vi "process safe state.vi"(8 "error in":errorcluster, 9 "result allocation":T1, 10 "parameters":T1, 11 "AppStateMachine runtime in":refnum<class "AppStateMachine runtime.lvclass">) -> (0 "error out":errorcluster, 1 "results":T1, 2 "parameter allocation":T1, 3 "AppStateMachine runtime out":refnum<class "AppStateMachine runtime.lvclass">)   [LabVIEW 2017, in "AppStateMachine runtime.lvclass"]
doc: "Provides an interface for information processing by a module when in a safe state. This interface simply calls the normal processing function. However, if child modules need to have custom logic during safe-state operation, this can be implemented here.\nNI Tag Bus Module Framework 1.0.2.34\nNI Systems Engineering"
uses:
  AppStateMachine runtime.lvclass
  <vilib>/NI/Tag Bus/table/data table.ctl
  State.ctl
  StateId.ctl
  LED_Color.ctl
  AppStateMachine runtime.lvclass/AppStateMachine runtime.ctl
  <vilib>/NI/Tag Bus/table/data table.lvlib
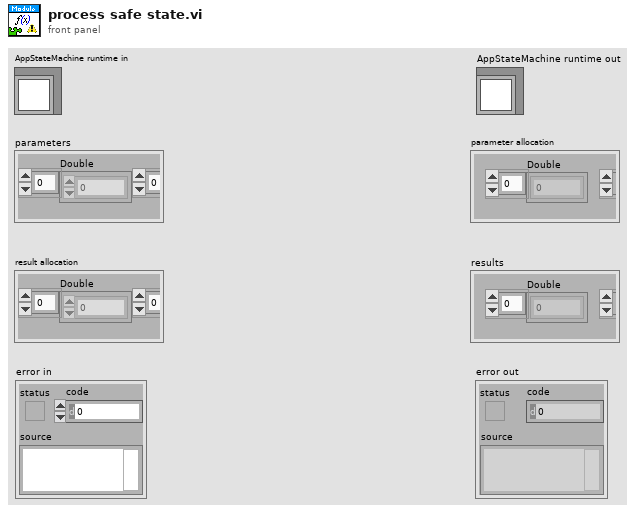
[diagram p1: front panel]
types:
  T1 = typedef "tag bus.lvlib/data table.lvlib/data table.ctl" = cluster{"Double":dbl[], "Single":sgl[], "I64":i64[], "I32":i32[], "I16":i16[], "I8":i8[], "U64":u64[], "U32":u32[], "U16":u16[], "U8":u8[], "Boolean":bool[], "String":string[], "Array of Double":cluster{"DBL Array":dbl[]}[], "Array of Single":cluster{"SGL Array":sgl[]}[], "Array of I64":cluster{"I64 Array":i64[]}[], "Array of I32":cluster{"I32 Array":i32[]}[], "Array of I16":cluster{"I16 Array":i16[]}[], "Array of I8":cluster{"I8 Array":i8[]}[], "Array of U64":cluster{"U64 Array":u64[]}[], "Array of U32":cluster{"U32 Array":u32[]}[], "Array of U16":cluster{"U16 Array":u16[]}[], "Array of U8":cluster{"U8 Array":u8[]}[], "Array of Boolean":cluster{"Boolean Array":bool[]}[], "Array of String":cluster{"String Array":string[]}[]}
  T2 = typedef "AppStateMachine runtime.lvclass/State.ctl" = cluster{"StateId":T3, "LED_Enable":bool, "LED_BlinksPerCycle":i32, "LED_Color":T4}
  T3 = typedef "AppStateMachine runtime.lvclass/StateId.ctl" = enum16{"Initialize", "Idle", "SafeState", "UnrecoverableSafeState"}
  T4 = typedef "AppStateMachine runtime.lvclass/LED_Color.ctl" = enum16{"Green", "Yellow"}
  T5 = typedef "AppStateMachine runtime.lvclass/result user data.ctl" = cluster{"State":u16, "LED_Enable":bool, "LED_BlinksPerCycle":i32, "LED_GreenOrYellow":bool}
  T6 = typedef "AppStateMachine configuration.lvclass/result data indices.ctl" = cluster{"U16.State":i32, "Boolean.LED_Enable":i32, "I32.LED_BlinksPerCycle":i32, "Boolean.LED_GreenOrYellow":i32}
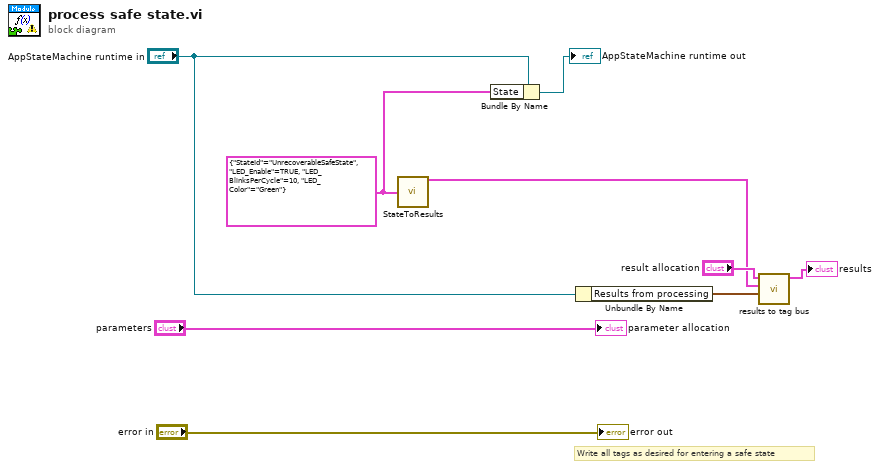
[diagram p0: block diagram]
diagram:
  w2 = T2 {"StateId"=enum."UnrecoverableSafeState", "LED_Enable"=TRUE, "LED_BlinksPerCycle"=10, "LED_Color"=enum."Green"} ("State")
  # "Write all tags as desired for entering a safe state"
  n1 = call "StateToResults.vi"("StateIn"=w2) -> ("Results"=w4:T5)  [unwired: 13 in, 1 out]
  n2 = Bundle By Name(cluster="AppStateMachine runtime in", "State"=w2) -> (→"AppStateMachine runtime out":refnum<class "AppStateMachine runtime.lvclass">)
  n3 = Unbundle By Name("AppStateMachine runtime in") -> ("Results from processing"=w7:T6)
  n4 = call "results to tag bus.vi"("indices"=w7, "data cluster"=w4, "tag bus in"="result allocation") -> ("tag bus out"=→"results":T1)  [unwired: 8 in]
  "error out" <- "error in"
  "parameter allocation" <- "parameters"
